vi "Кластеры-03-масштабирование.vi"() -> ()   [LabVIEW 2017]
doc: "Exercise 5-6 of the LabVIEW Basics I course\nThis VI illustrates the use of polymorphism to operate on a cluster of numeric information. Most of LabVIEW's built in functions can operate on many different data structures. For example, you can use the sin(x) function on any kind of numeric data, be it a scalar number, an n-dimensional array fo numbers, or an arbitrarily complex cluster of numeric data.\n\nPolymorphism keeps your VI diagrams smaller and easier to understand, and simplifies your programming."
panel:
  out "Масштабированные данные":T1 {"Давление (Н/м^2)" scale=1000.0..100000.0; "Расход (литры/сек)" scale=0.0..100.0; "Температура(град.C)" scale=0.0..500.0}
  in  "Входные данные":T2 {"В (давление)" format="%.2f"; "В (расход)" format="%.2f"; "В (температура)" format="%.2f"}
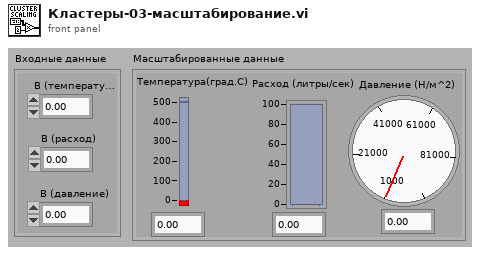
[diagram p1: front panel]
types:
  T1 = cluster{"Температура(град.C)":dbl, "Расход (литры/сек)":dbl, "Давление (Н/м^2)":dbl}
  T2 = cluster{"В (температура)":dbl, "В (расход)":dbl, "В (давление)":dbl}
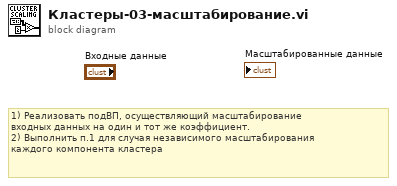
[diagram p0: block diagram]
diagram:
  # "1) Реализовать подВП, осуществляющий масштабирование \nвходных данных на один и тот же коэффициент.\n2) Выполнить п.1 для случая независимого масштабирования \nкаждого компонента кластера"
